vi "Copy Client Template Library.vi"(8 "error in":errorcluster, 10 "new library name":string, 11 "project ref":refnum<vi>) -> (0 "error out":errorcluster, 3 "file refnums":refnum<vi>[](array[refnum]))   [LabVIEW 2021, in "NI Measurement V2 Client Generator Runtime.lvlib"]
uses:
  NI Measurement V2 Client Generator Runtime.lvlib
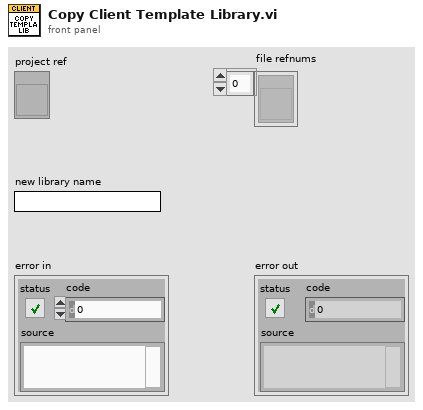
[diagram p1: front panel]
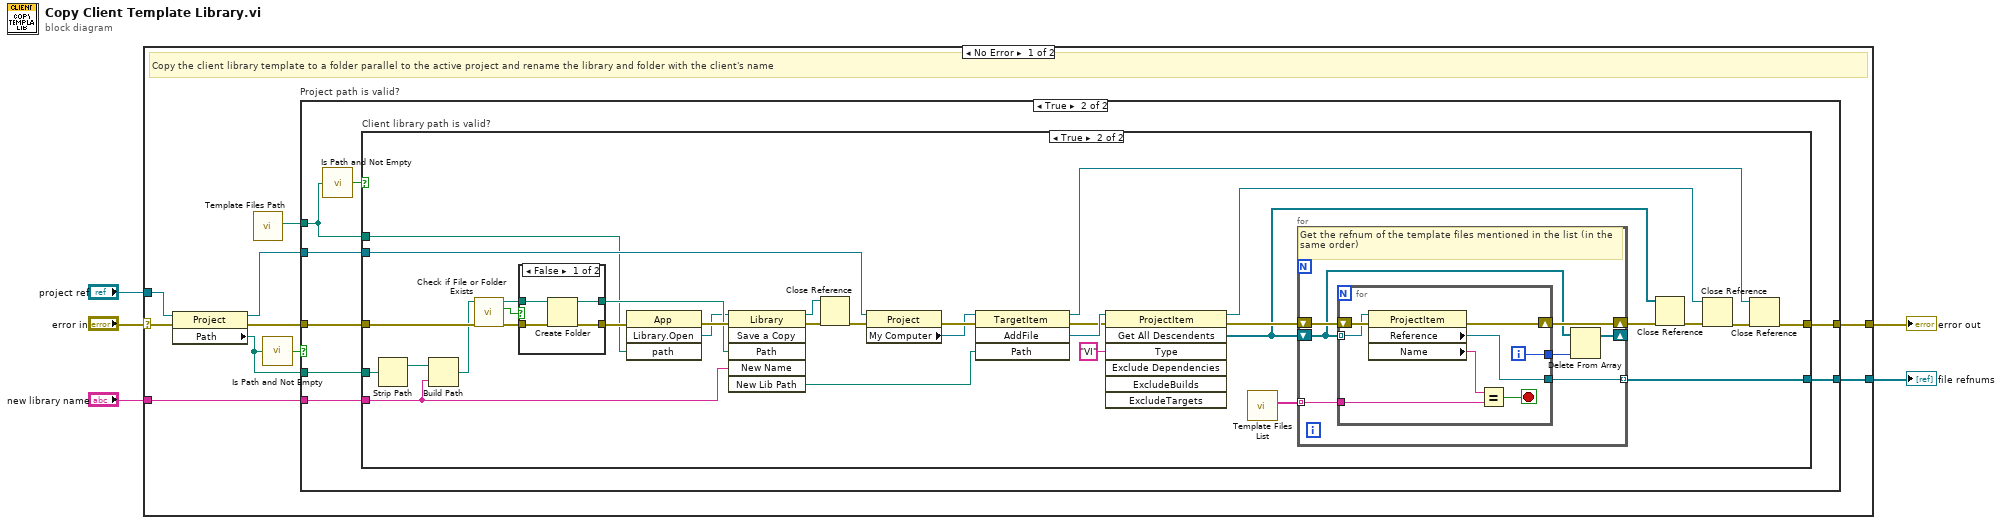
[diagram p0: block diagram]
diagram:
  n1 = case shown="No Error" "error in" {
    selector: "error in" -> [w13 w80]
    tunnel: "project ref" -> [w15 _]
    tunnel: "new library name" -> [w10 _]
    tunnel: [w8 w80] -> w2
    tunnel: [w7 _] -> w1
    frame No Error {
      # "Copy the client library template to a folder parallel to the active project and rename the library and folder with the client's name"
      n2 = property class="Project"(reference=w15, error in=w13) -> (reference out=w9:refnum<vi>, error out=w14:errorcluster, "Path"=w11:path)
      n3 = call "Template Files Path.vi"() -> ("template lib path"=w6:path)  [unwired: 9 in, 2 out]
      n4 = call <vilib>:"Is Path and Not Empty.vi"("path"=w11) -> ("Is Path and Not Empty?"=w12:bool)  [unwired: 4 in]
      n5 = case "Project path is valid?" shown="True" w12 {
        tunnel: w14 -> [w16 w24]
        tunnel: w6 -> [_ w19]
        tunnel: w11 -> [_ w23]
        tunnel: w10 -> [_ w22]
        tunnel: w9 -> [_ w21]
        tunnel: [w16 w20] -> w8
        tunnel: [_ w17] -> w7
        frame False {
        }
        frame True {
          n6 = call <vilib>:"Is Path and Not Empty.vi"("path"=w19) -> ("Is Path and Not Empty?"=w18:bool)  [unwired: 4 in]
          n7 = case "Client library path is valid?" shown="True" w18 {
            tunnel: w24 -> [w25 w58]
            tunnel: w23 -> [_ w56]
            tunnel: w22 -> [_ w48]
            tunnel: w21 -> [_ w46]
            tunnel: [w25 w33] -> w20
            tunnel: w19 -> [_ w31]
            tunnel: [_ w29] -> w17
            frame False {
            }
            frame True {
              n8 = Strip Path(path=w56) -> (stripped path=w55:path)  [unwired: 1 out]
              n9 = Build Path(base path=w55, name or relative path=w48) -> (appended path=w54:path)
              n10 = call <vilib>:"Check if File or Folder Exists.vi"("error in (no error)"=w58, "path"=w54) -> ("error out"=w53:errorcluster, "file or folder exists?"=w52:bool, "dup path"=w51:path)  [unwired: 7 in]
              n11 = case shown="False" w52 {
                tunnel: w53 -> [w77 w78]
                tunnel: w51 -> [w76 w79]
                tunnel: [w75 w78] -> w49
                tunnel: [w74 w79] -> w50
                frame False {
                  n12 = Create Folder(path (use dialog)=w76, error in=w77) -> (created path=w74:path, error out=w75:errorcluster)  [unwired: 1 in, 1 out]
                }
                frame True {
                }
              }
              n13 = invoke class="App" method="Library.Open"(error in=w49, "path"=w31) -> (error out=w57:errorcluster, "Open Library"=w47:refnum<vi>)  [unwired: 2 in, 2 out]
              n14 = invoke class="Library" method="Save a Copy"(reference=w47, error in=w57, "Path"=w50, "New Name"=w48) -> (reference out=w43:refnum<vi>, error out=w44:errorcluster, "New Lib Path"=w41:path)  [unwired: 2 in, 3 out]
              n15 = Close Reference(reference=w43, error in (no error)=w44) -> (error out=w45:errorcluster)
              n16 = property class="Project"(reference=w46, error in=w45) -> (error out=w42:errorcluster, "My Computer"=w32:refnum<vi>)  [unwired: 1 out]
              n17 = invoke class="TargetItem" method="AddFile"(reference=w32, error in=w42, "Path"=w41) -> (reference out=w35:refnum<vi>, error out=w39:errorcluster, "AddFile"=w40:refnum<vi>)  [unwired: 1 in, 1 out]
              n18 = invoke class="ProjectItem" method="Get All Descendents"(reference=w40, error in=w39, "Type"="VI") -> (reference out=w34:refnum<vi>, error out=w37:errorcluster, "All Descendents"=w27:refnum<vi>[])  [unwired: 4 in, 4 out]
              n19 = call "Template Files List.vi"() -> ("template files"=w26:string[])  [unwired: 11 in]
              n20 = for {
                tunnel: [w64] -> w29 mode=indexing
                shift-right: [w60] -> w30
                shift-left: w37 -> [w65]
                tunnel: w26 -> [w63] mode=indexing
                shift-right: [w61] -> _
                shift-left: w27 -> [w59]
                # "Get the refnum of the template files mentioned in the list (in the same order)"
                n21 = for {
                  tunnel: w59 -> [w72] mode=indexing
                  tunnel: [w71] -> w64
                  tunnel: w63 -> [w69]
                  tunnel: [w68] -> w62
                  shift-right: [w66] -> w60
                  shift-left: w65 -> [w73]
                  i -> [w68]
                  stop <- w67 stop-if-true
                  # "Get references of controls and VIs to be modified"
                  n22 = property class="ProjectItem"(reference=w72, error in=w73) -> (error out=w66:errorcluster, "Reference"=w71:refnum<vi>, "Name"=w70:string)  [unwired: 1 out]
                  n23 = Equal?(x=w70, y=w69) -> (x = y?=w67:bool)
                }
                n24 = Delete From Array(array=w59, index=w62) -> (array with subset deleted=w61:refnum<vi>[])  [unwired: 1 in, 1 out]
              }
              n25 = Close Reference(reference=w27, error in (no error)=w30) -> (error out=w28:errorcluster)
              n26 = Close Reference(reference=w34, error in (no error)=w28) -> (error out=w36:errorcluster)
              n27 = Close Reference(reference=w35, error in (no error)=w36) -> (error out=w33:errorcluster)
            }
          }
        }
      }
    }
    frame Error {
      # "Pass"
    }
  }
  "error out" <- w2
  "file refnums" <- w1
